vi "Correct Taus.vi"(4 "#_shots":i32=5, 6 "Filter?":bool, 8 "error in":errorcluster, 9 "filter changed?":bool, 11 "CRDS Cell in":refnum<class "CRDS Cell.lvclass">) -> (0 "error out":errorcluster, 3 "CRDS Cell out":refnum<class "CRDS Cell.lvclass">)   [LabVIEW 2018, in "CRDS Lib.lvlib" / "CRDS Cell.lvclass"]
doc: "Correct tau values for Rayleigh scattering. \n\nIf on filter:\n* The tau and tau0 values will be the uncorrected values in seconds.\n* tau0corr will be in the Rayleigh scattering corrected value in us.\n* ext, extcorr and taucorr will be set to NaN.\n\nIf on sample:\n* Tau is the raw tau value in us.\n* taucorr will be the Rayleigh scattering corrected value in us\n* ext and extCorr will be the same value."
uses:
  CRDS Cell.lvclass
  CRDS Cell.lvclass/CRDS Cell.ctl
  Data/Cell/CRDS Cell Data.lvclass/CRDS Cell Data.ctl
  Data/Cell/Read extParam.vi
  Data/Cell/Read hkParam.vi
  General/Atmospheric/Atmospheric Constants.vi
  General/Atmospheric/Atmospheric Library.lvlib
  Data/Cell/CRDS Cell Data.lvclass
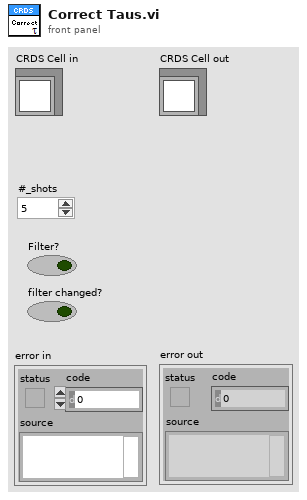
[diagram p1: front panel]
types:
  T1 = typedef "Base CRDS Lib.lvlib/calData.ctl" = cluster{"rhDilFac":sgl, "Q":sgl, "Tmean":sgl, "extDilFac":sgl, "rhCell":sgl, "P":sgl, "T":sgl}
  T2 = typedef "extparam.ctl" = cluster{"Tau":sgl, "Tau0cor":sgl, "ext":sgl, "extCorr":sgl, "stdevTau":sgl, "eTau":sgl, "taucorr":sgl, "Tau0":sgl, "max":sgl}
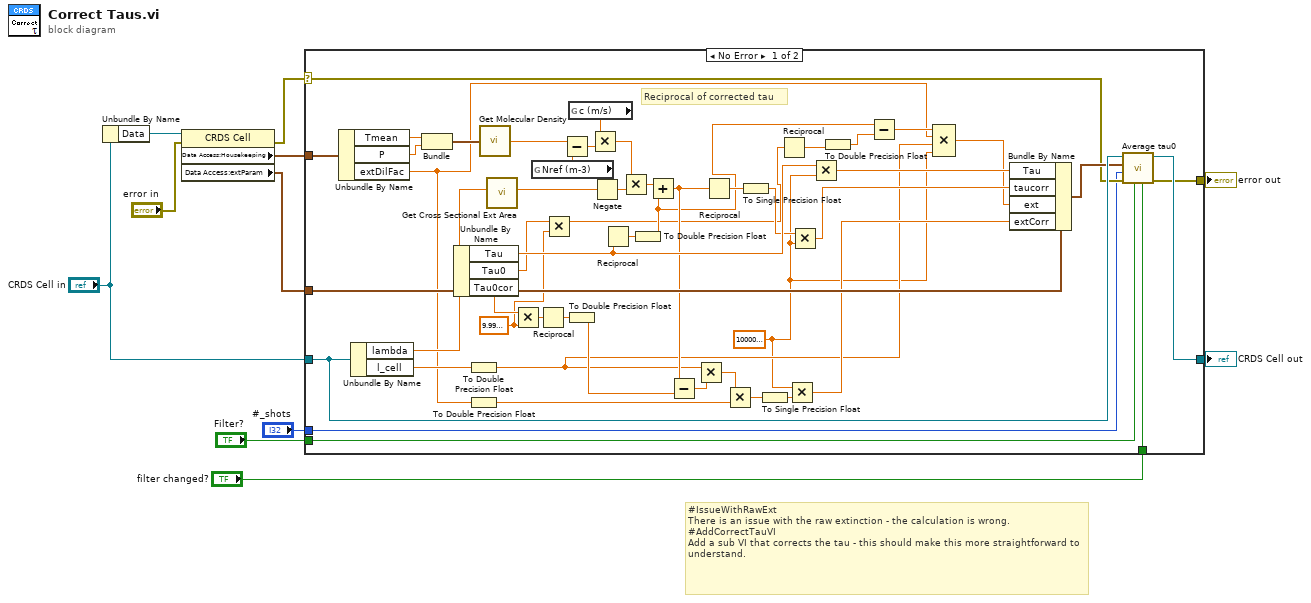
[diagram p0: block diagram]
diagram:
  # "#IssueWithRawExt\nThere is an issue with the raw extinction - the calculation is wrong.\n#AddCorrectTauVI\nAdd a sub VI that corrects the tau - this should make this more straightforward to understand."
  n1 = Unbundle By Name("CRDS Cell in") -> ("Data"=w4:refnum<class "CRDS Cell Data.lvclass">)
  n2 = property class="CRDS Cell"(reference=w4, error in="error in") -> (error out=w6:errorcluster, "Data Access:Housekeeping"=w9:T1, "Data Access:extParam"=w8:T2)  [unwired: 1 out]
  n3 = case shown="No Error" w6 {
    selector: w6 -> [w53 w64]
    tunnel: [w52 w64] -> w3
    tunnel: [w55 w63] -> w2
    tunnel: "CRDS Cell in" -> [w56 w63]
    tunnel: w9 -> [w62 _]
    tunnel: w8 -> [w60 _]
    tunnel: "Filter?" -> [w33 _]
    tunnel: "#_shots" -> [w51 _]
    tunnel: "filter changed?" -> [w50 _]
    frame No Error {
      w12 = sgl 1e-06
      w15 = sgl 1000000.0
      # "Reciprocal of corrected tau"
      n4 = Unbundle By Name(w62) -> ("Tmean"=w61:sgl, "P"=w57:sgl, "extDilFac"=w18:sgl)
      n5 = Unbundle By Name(w56) -> ("lambda"=w58:dbl, "l_cell"=w59:sgl)
      n6 = Bundle("Tmean"=w61, "P"=w57) -> (w31:cluster{"Tmean":sgl, "P":sgl})  [unwired: 1 in]
      n7 = Unbundle By Name(w60) -> ("Tau"=w45:sgl, "Tau0"=w19:sgl, "Tau0cor"=w23:sgl)
      n8 = To Double Precision Float(number=w59) -> (double precision float=w17:dbl)
      n9 = To Double Precision Float(number=w18) -> (double precision float=w26:dbl)
      n10 = call "Get Molecular Density.vi"("thermoCond"=w31) -> ("M (m-3)"=w32:dbl)
      n11 = call "Get Cross Sectional Ext Area.vi"("l (nm)"=w58) -> ("CAext (m2)"=w30:dbl)  [unwired: 10 in]
      n12 = Multiply(x=w23, y=w12) -> (x*y=w34:sgl)
      n13 = global read "Atmospheric Constants.vi" "Nref (m-3)"() -> (w49:dbl)
      n14 = Reciprocal(x=w34) -> (1/x=w35:sgl)
      n15 = Multiply(x=w19, y=w12) -> (x*y=w13:sgl)
      n16 = Subtract(x=w32, y=w49) -> (x-y=w44:dbl)
      n17 = To Double Precision Float(number=w35) -> (double precision float=w27:dbl)
      n18 = global read "Atmospheric Constants.vi" "c (m/s)"() -> (w43:dbl)
      n19 = Multiply(x=w43, y=w44) -> (x*y=w48:dbl)
      n20 = Negate(x=w30) -> (-x=w29:dbl)
      n21 = Reciprocal(x=w45) -> (1/x=w47:sgl)
      n22 = Multiply(x=w48, y=w29) -> (x*y=w28:dbl)
      n23 = To Double Precision Float(number=w47) -> (double precision float=w14:dbl)
      n24 = Add(x=w28, y=w14) -> (x+y=w37:dbl)
      n25 = Subtract(x=w37, y=w27) -> (x-y=w41:dbl)
      n26 = Multiply(x=w17, y=w41) -> (x*y=w38:dbl)
      n27 = Reciprocal(x=w37) -> (1/x=w36:dbl)
      n28 = Multiply(x=w38, y=w26) -> (x*y=w40:dbl)
      n29 = To Single Precision Float(number=w36) -> (single precision float=w42:sgl)
      n30 = To Single Precision Float(number=w40) -> (single precision float=w39:sgl)
      n31 = Reciprocal(x=w13) -> (1/x=w22:sgl)
      n32 = Multiply(x=w15, y=w39) -> (x*y=w24:sgl)
      n33 = Multiply(x=w42, y=w15) -> (x*y=w25:sgl)
      n34 = Multiply(x=w45, y=w15) -> (x*y=w46:sgl)
      n35 = To Double Precision Float(number=w22) -> (double precision float=w21:dbl)
      n36 = Subtract(x=w14, y=w21) -> (x-y=w20:dbl)
      n37 = Compound Arithmetic op=MULTIPLY(w20, w18, w17, w15) -> (w16:dbl)
      n38 = Bundle By Name(cluster=w60, "Tau"=w46, "taucorr"=w25, "ext"=w16, "extCorr"=w24) -> (w54:T2)
      n39 = call "Average tau0.vi"("filter changed?"=w50, "filter"=w33, "error in"=w53, "# of shots"=w51, "extParam"=w54, "CRDS Cell in"=w56) -> ("error out"=w52:errorcluster, "CRDS Cell out"=w55:refnum<class "CRDS Cell.lvclass">)  [unwired: 4 in]
    }
    frame Error {
    }
  }
  "error out" <- w3
  "CRDS Cell out" <- w2
